vi "Write Settings 2.vi"(8 "error in (no error)":errorcluster, 10 "Settings":T1={"Trigger"=enum."off", "Gain"={"Value"=0.0, "Min"=0.0, "Max"=12.0, "StepSize"=0.1, "Tolerance"=0.0, "valueactual"=0.0}, "Exposure"={"Value"=0.001, "Min"=3.8e-05, "Max"=1.0, "StepSize"=1e-06, "Tolerance"=0.0, "valueactual"=0.0}, "Timeout"={"Value"=5000.0, "Min"=100.0, "Max"=5000.0, "StepSize"=100.0, "Tolerance"=0.0, "valueactual"=0.0}, "LocalSavingPath"=path "c:/temp", "Save"=enum."off", "TriggerDelay"={"Value"=0.0, "Min"=0.0, "Max"=0.09, "StepSize"=0.001, "Tolerance"=0.0, "valueactual"=0.0}, "CamSession"="cam2", "ROI"={"Width"={"Value"=618.0, "Min"=1.0, "Max"=3000.0, "StepSize"=1.0, "Tolerance"=0.0, "valueactual"=0.0}, "Height"={"Value"=813.0, "Min"=1.0, "Max"=3000.0, "StepSize"=1.0, "Tolerance"=0.0, "valueactual"=0.0}, "OffsetX"={"Value"=0.0, "Min"=0.0, "Max"=1000.0, "StepSize"=1.0, "Tolerance"=0.0, "valueactual"=0.0}, "OffsetY"={"Value"=0.0, "Min"=0.0, "Max"=1000.0, "StepSize"=1.0, "Tolerance"=0.0, "valueactual"=0.0}}, "MaxGUIPixel"={"Value"=2000.0, "Min"=10.0, "Max"=2000.0, "StepSize"=10.0, "Tolerance"=0.0, "valueactual"=0.0}, "Target"={"X"={"Value"=200.0, "Min"=0.0, "Max"=2000.0, "StepSize"=1.0, "Tolerance"=0.0, "valueactual"=0.0}, "Y"={"Value"=200.0, "Min"=0.0, "Max"=2000.0, "StepSize"=1.0, "Tolerance"=0.0, "valueactual"=0.0}}, "Analysis"=enum."off", "maxshot#"=10000.0, "SpatialCalibration"={"Value"=1.0, "Min"=0.0, "Max"=99999999.0, "StepSize"=0.001, "Tolerance"=0.0, "valueactual"=0.0}, "roistatus"=enum."on", "Lineout"=enum."off", "AnalysisThreshold"={"Value"=0.9, "Min"=0.0, "Max"=3000.0, "StepSize"=0.1, "Tolerance"=0.0, "valueactual"=0.0}, "TargetSize"={"X"={"Value"=200.0, "Min"=0.0, "Max"=2000.0, "StepSize"=1.0, "Tolerance"=0.0, "valueactual"=0.0}, "Y"={"Value"=200.0, "Min"=0.0, "Max"=2000.0, "StepSize"=1.0, "Tolerance"=0.0, "valueactual"=0.0}}, "Simulation"=enum."off", "SpatialCalibrationY"={"Value"=1.0, "Min"=0.0, "Max"=99999999.0, "StepSize"=0.001, "Tolerance"=0.0, "valueactual"=0.0}, "Target2"={"X"={"Value"=200.0, "Min"=0.0, "Max"=2000.0, "StepSize"=1.0, "Tolerance"=0.0, "valueactual"=0.0}, "Y"={"Value"=200.0, "Min"=0.0, "Max"=2000.0, "StepSize"=1.0, "Tolerance"=0.0, "valueactual"=0.0}}, "Target2Size"={"X"={"Value"=200.0, "Min"=0.0, "Max"=2000.0, "StepSize"=1.0, "Tolerance"=0.0, "valueactual"=0.0}, "Y"={"Value"=200.0, "Min"=0.0, "Max"=2000.0, "StepSize"=1.0, "Tolerance"=0.0, "valueactual"=0.0}}, "Crosshair"={"Label1"="", "Label2"=""}, "Max2ndMomRadius"={"Value"=100.0, "Min"=0.0, "Max"=3000.0, "StepSize"=10.0, "Tolerance"=0.0, "valueactual"=0.0}, "SaveType"=enum."PNG", "BackgroundPath"=path "", "GUI8bit"=enum."on", "GUICompression"=enum."on", "CompressionQuality"={"Value"=1000.0, "Min"=0.0, "Max"=1000.0, "StepSize"=1.0, "Tolerance"=1.0, "valueactual"=0.0}, "SaveAsync"=enum."off", "PerspectivePath"=path "", "PerspectiveCorrectGUI"=enum."off", "BlackLevel"={"Value"=0.0, "Min"=0.0, "Max"=3.0, "StepSize"=0.001, "Tolerance"=0.0, "valueactual"=0.0}, "TargetBP"={"X"={"Value"=200.0, "Min"=0.0, "Max"=2000.0, "StepSize"=1.0, "Tolerance"=0.0, "valueactual"=0.0}, "Y"={"Value"=200.0, "Min"=0.0, "Max"=2000.0, "StepSize"=1.0, "Tolerance"=0.0, "valueactual"=0.0}}, "PythonAnalysis"=enum."off", "PythonFunctionName"="cam2", "PythonLineout"=enum."off", "PythonVersion"="cam2", "GEECSBuildsPath"=path "", "DisplayPythonProcessedImage"=enum."off", "PythonModuleName"="cam2", "AnalysisThresholdHigh"={"Value"=0.9, "Min"=0.0, "Max"=3000.0, "StepSize"=0.1, "Tolerance"=0.0, "valueactual"=0.0}, "AnalysisMedianRank"={"Value"=0.0, "Min"=0.0, "Max"=0.0, "StepSize"=0.0, "Tolerance"=0.0, "valueactual"=0.0}, "ClockSpeed"={"Value"=4094.0, "Min"=0.0, "Max"=65000.0, "StepSize"=1.0, "Tolerance"=0.0, "valueactual"=0.0}, "AutoTrigger"=enum."off", "AutoTriggerLevelMeanCounts"={"Value"=0.0, "Min"=0.0, "Max"=3.0, "StepSize"=0.001, "Tolerance"=0.0, "valueactual"=0.0}, "AnalysisROILeft"={"Value"=0.0, "Min"=0.0, "Max"=0.0, "StepSize"=0.0, "Tolerance"=0.0, "valueactual"=0.0}, "AnalysisROIRight"={"Value"=0.0, "Min"=0.0, "Max"=0.0, "StepSize"=0.0, "Tolerance"=0.0, "valueactual"=0.0}, "AnalysisROITop"={"Value"=0.0, "Min"=0.0, "Max"=0.0, "StepSize"=0.0, "Tolerance"=0.0, "valueactual"=0.0}, "AnalysisROIBottom"={"Value"=0.0, "Min"=0.0, "Max"=0.0, "StepSize"=0.0, "Tolerance"=0.0, "valueactual"=0.0}, "AnalysisROI"=enum."off", "UseSoftwareTrigger"=enum."off", "UDPtrigger"=enum."off", "AutoTriggerLevelMaxCounts"={"Value"=0.0, "Min"=0.0, "Max"=3.0, "StepSize"=0.001, "Tolerance"=0.0, "valueactual"=0.0}}, 11 "Point Grey Camera in":refnum<class "Point Grey Camera.lvclass">) -> (0 "error out":errorcluster, 3 "Point Grey Camera out":refnum<class "Point Grey Camera.lvclass">)   [LabVIEW 2020, in "Point Grey Camera.lvclass"]
uses:
  Point Grey Camera.lvclass
  SettingsTypdef.ctl
  shared/OnOffTypeDef.ctl
  subVis/ROI_TypDef.ctl
  subVis/Image save type.ctl
  Point Grey Camera.lvclass/Point Grey Camera.ctl
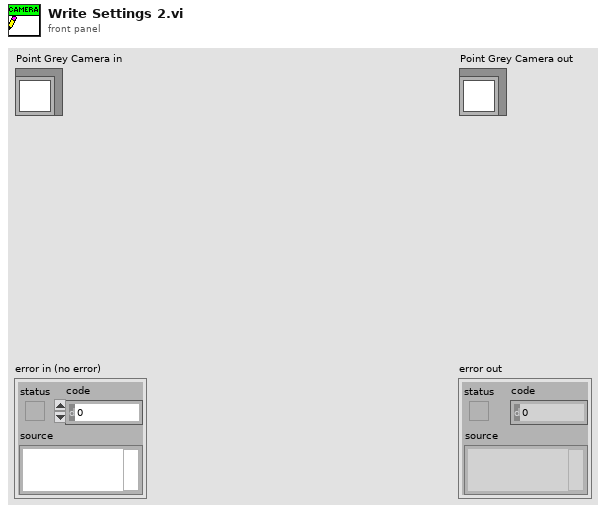
[diagram p1: front panel]
types:
  T1 = typedef "Point Grey Camera.lvclass/SettingsTypdef.ctl" = cluster{"Trigger":T2, "Gain":cluster{"Value":dbl, "Min":dbl, "Max":dbl, "StepSize":dbl, "Tolerance":dbl, "valueactual":dbl}, "Exposure":cluster{"Value":dbl, "Min":dbl, "Max":dbl, "StepSize":dbl, "Tolerance":dbl, "valueactual":dbl}, "Timeout":cluster{"Value":dbl, "Min":dbl, "Max":dbl, "StepSize":dbl, "Tolerance":dbl, "valueactual":dbl}, "LocalSavingPath":path, "Save":T2, "TriggerDelay":cluster{"Value":dbl, "Min":dbl, "Max":dbl, "StepSize":dbl, "Tolerance":dbl, "valueactual":dbl}, "CamSession":string, "ROI":T3, "MaxGUIPixel":cluster{"Value":dbl, "Min":dbl, "Max":dbl, "StepSize":dbl, "Tolerance":dbl, "valueactual":dbl}, "Target":cluster{"X":cluster{"Value":dbl, "Min":dbl, "Max":dbl, "StepSize":dbl, "Tolerance":dbl, "valueactual":dbl}, "Y":cluster{"Value":dbl, "Min":dbl, "Max":dbl, "StepSize":dbl, "Tolerance":dbl, "valueactual":dbl}}, "Analysis":T2, "maxshot#":dbl, "SpatialCalibration":cluster{"Value":dbl, "Min":dbl, "Max":dbl, "StepSize":dbl, "Tolerance":dbl, "valueactual":dbl}, "roistatus":T2, "Lineout":T2, "AnalysisThreshold":cluster{"Value":dbl, "Min":dbl, "Max":dbl, "StepSize":dbl, "Tolerance":dbl, "valueactual":dbl}, "TargetSize":cluster{"X":cluster{"Value":dbl, "Min":dbl, "Max":dbl, "StepSize":dbl, "Tolerance":dbl, "valueactual":dbl}, "Y":cluster{"Value":dbl, "Min":dbl, "Max":dbl, "StepSize":dbl, "Tolerance":dbl, "valueactual":dbl}}, "Simulation":T2, "SpatialCalibrationY":cluster{"Value":dbl, "Min":dbl, "Max":dbl, "StepSize":dbl, "Tolerance":dbl, "valueactual":dbl}, "Target2":cluster{"X":cluster{"Value":dbl, "Min":dbl, "Max":dbl, "StepSize":dbl, "Tolerance":dbl, "valueactual":dbl}, "Y":cluster{"Value":dbl, "Min":dbl, "Max":dbl, "StepSize":dbl, "Tolerance":dbl, "valueactual":dbl}}, "Target2Size":cluster{"X":cluster{"Value":dbl, "Min":dbl, "Max":dbl, "StepSize":dbl, "Tolerance":dbl, "valueactual":dbl}, "Y":cluster{"Value":dbl, "Min":dbl, "Max":dbl, "StepSize":dbl, "Tolerance":dbl, "valueactual":dbl}}, "Crosshair":cluster{"Label1":string, "Label2":string}, "Max2ndMomRadius":cluster{"Value":dbl, "Min":dbl, "Max":dbl, "StepSize":dbl, "Tolerance":dbl, "valueactual":dbl}, "SaveType":T4, "BackgroundPath":path, "GUI8bit":T2, "GUICompression":T2, "CompressionQuality":cluster{"Value":dbl, "Min":dbl, "Max":dbl, "StepSize":dbl, "Tolerance":dbl, "valueactual":dbl}, "SaveAsync":T2, "PerspectivePath":path, "PerspectiveCorrectGUI":T2, "BlackLevel":cluster{"Value":dbl, "Min":dbl, "Max":dbl, "StepSize":dbl, "Tolerance":dbl, "valueactual":dbl}, "TargetBP":cluster{"X":cluster{"Value":dbl, "Min":dbl, "Max":dbl, "StepSize":dbl, "Tolerance":dbl, "valueactual":dbl}, "Y":cluster{"Value":dbl, "Min":dbl, "Max":dbl, "StepSize":dbl, "Tolerance":dbl, "valueactual":dbl}}, "PythonAnalysis":T2, "PythonFunctionName":string, "PythonLineout":T2, "PythonVersion":string, "GEECSBuildsPath":path, "DisplayPythonProcessedImage":T2, "PythonModuleName":string, "AnalysisThresholdHigh":cluster{"Value":dbl, "Min":dbl, "Max":dbl, "StepSize":dbl, "Tolerance":dbl, "valueactual":dbl}, "AnalysisMedianRank":cluster{"Value":dbl, "Min":dbl, "Max":dbl, "StepSize":dbl, "Tolerance":dbl, "valueactual":dbl}, "ClockSpeed":cluster{"Value":dbl, "Min":dbl, "Max":dbl, "StepSize":dbl, "Tolerance":dbl, "valueactual":dbl}, "AutoTrigger":T2, "AutoTriggerLevelMeanCounts":cluster{"Value":dbl, "Min":dbl, "Max":dbl, "StepSize":dbl, "Tolerance":dbl, "valueactual":dbl}, "AnalysisROILeft":cluster{"Value":dbl, "Min":dbl, "Max":dbl, "StepSize":dbl, "Tolerance":dbl, "valueactual":dbl}, "AnalysisROIRight":cluster{"Value":dbl, "Min":dbl, "Max":dbl, "StepSize":dbl, "Tolerance":dbl, "valueactual":dbl}, "AnalysisROITop":cluster{"Value":dbl, "Min":dbl, "Max":dbl, "StepSize":dbl, "Tolerance":dbl, "valueactual":dbl}, "AnalysisROIBottom":cluster{"Value":dbl, "Min":dbl, "Max":dbl, "StepSize":dbl, "Tolerance":dbl, "valueactual":dbl}, "AnalysisROI":T2, "UseSoftwareTrigger":T2, "UDPtrigger":T2, "AutoTriggerLevelMaxCounts":cluster{"Value":dbl, "Min":dbl, "Max":dbl, "StepSize":dbl, "Tolerance":dbl, "valueactual":dbl}}
  T2 = typedef "OnOffTypeDef.ctl" = enum16{"off", "on"}
  T3 = typedef "ROI_TypDef.ctl" = cluster{"Width":cluster{"Value":dbl, "Min":dbl, "Max":dbl, "StepSize":dbl, "Tolerance":dbl, "valueactual":dbl}, "Height":cluster{"Value":dbl, "Min":dbl, "Max":dbl, "StepSize":dbl, "Tolerance":dbl, "valueactual":dbl}, "OffsetX":cluster{"Value":dbl, "Min":dbl, "Max":dbl, "StepSize":dbl, "Tolerance":dbl, "valueactual":dbl}, "OffsetY":cluster{"Value":dbl, "Min":dbl, "Max":dbl, "StepSize":dbl, "Tolerance":dbl, "valueactual":dbl}}
  T4 = typedef "Image save type.ctl" = enum16{"PNG", "BMP", "JPEG", "TDMS", "hdf5"}
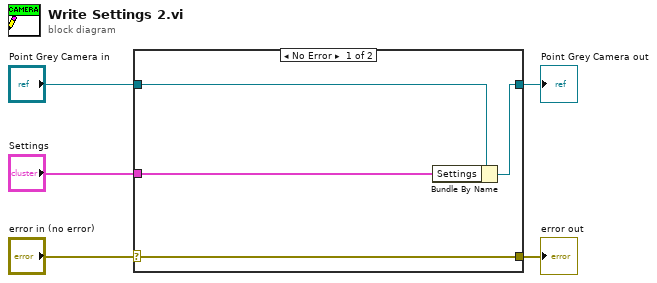
[diagram p0: block diagram]
diagram:
  n1 = case shown="No Error" "error in (no error)" {
    selector: "error in (no error)" -> [w9 w10]
    tunnel: [w9 w10] -> w4
    tunnel: [w7 w11] -> w2
    tunnel: "Point Grey Camera in" -> [w8 w11]
    tunnel: "Settings" -> [w6 _]
    frame No Error {
      n2 = Bundle By Name(cluster=w8, "Settings"=w6) -> (w7:refnum<class "Point Grey Camera.lvclass">)
    }
    frame Error {
    }
  }
  "error out" <- w4
  "Point Grey Camera out" <- w2
